vi "PAQ_FileRef_read_all_samples.vi"(8 "error in (no error)":errorcluster, 11 "refnum in":refnum<file>) -> (0 "error out":errorcluster, 1 "data":T1, 2 "Fetched samples":i32, 3 "refnum out":refnum<file>)   [LabVIEW 2020, in "Sgraph_lib_V1.lvlib" / "DBAL-BIN.lvclass"]
doc: "Read all samples from one PAQ file based on a file reference.\nThis VI will leave the file open, with the pointer right where the first data should be saved.\nPurpose is to replace the whole file content with a new data portion added.\nIn this way a file concatenate action without segmentation is performed."
uses:
  DBAL-BIN.lvclass
  controls/BIN/BINdata.ctl
panel:
  out "TAGs":string[](array[string])
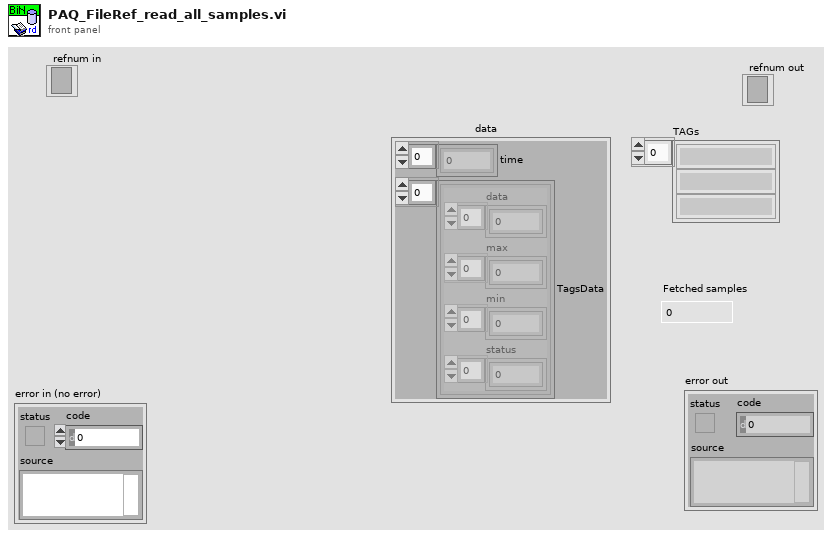
[diagram p1: front panel]
types:
  T1 = typedef "Sgraph_lib_V1.lvlib/DBAL-BIN.lvclass/BINdata.ctl" = cluster{"time":dbl[], "TagsData":cluster{"data":dbl[], "max":dbl[], "min":dbl[], "status":u32[]}[]}
  T2 = cluster{"data":dbl[], "max":dbl[], "min":dbl[], "status":u32[]}[]
  T3 = cluster{"data":dbl[], "max":dbl[], "min":dbl[], "status":u32[]}
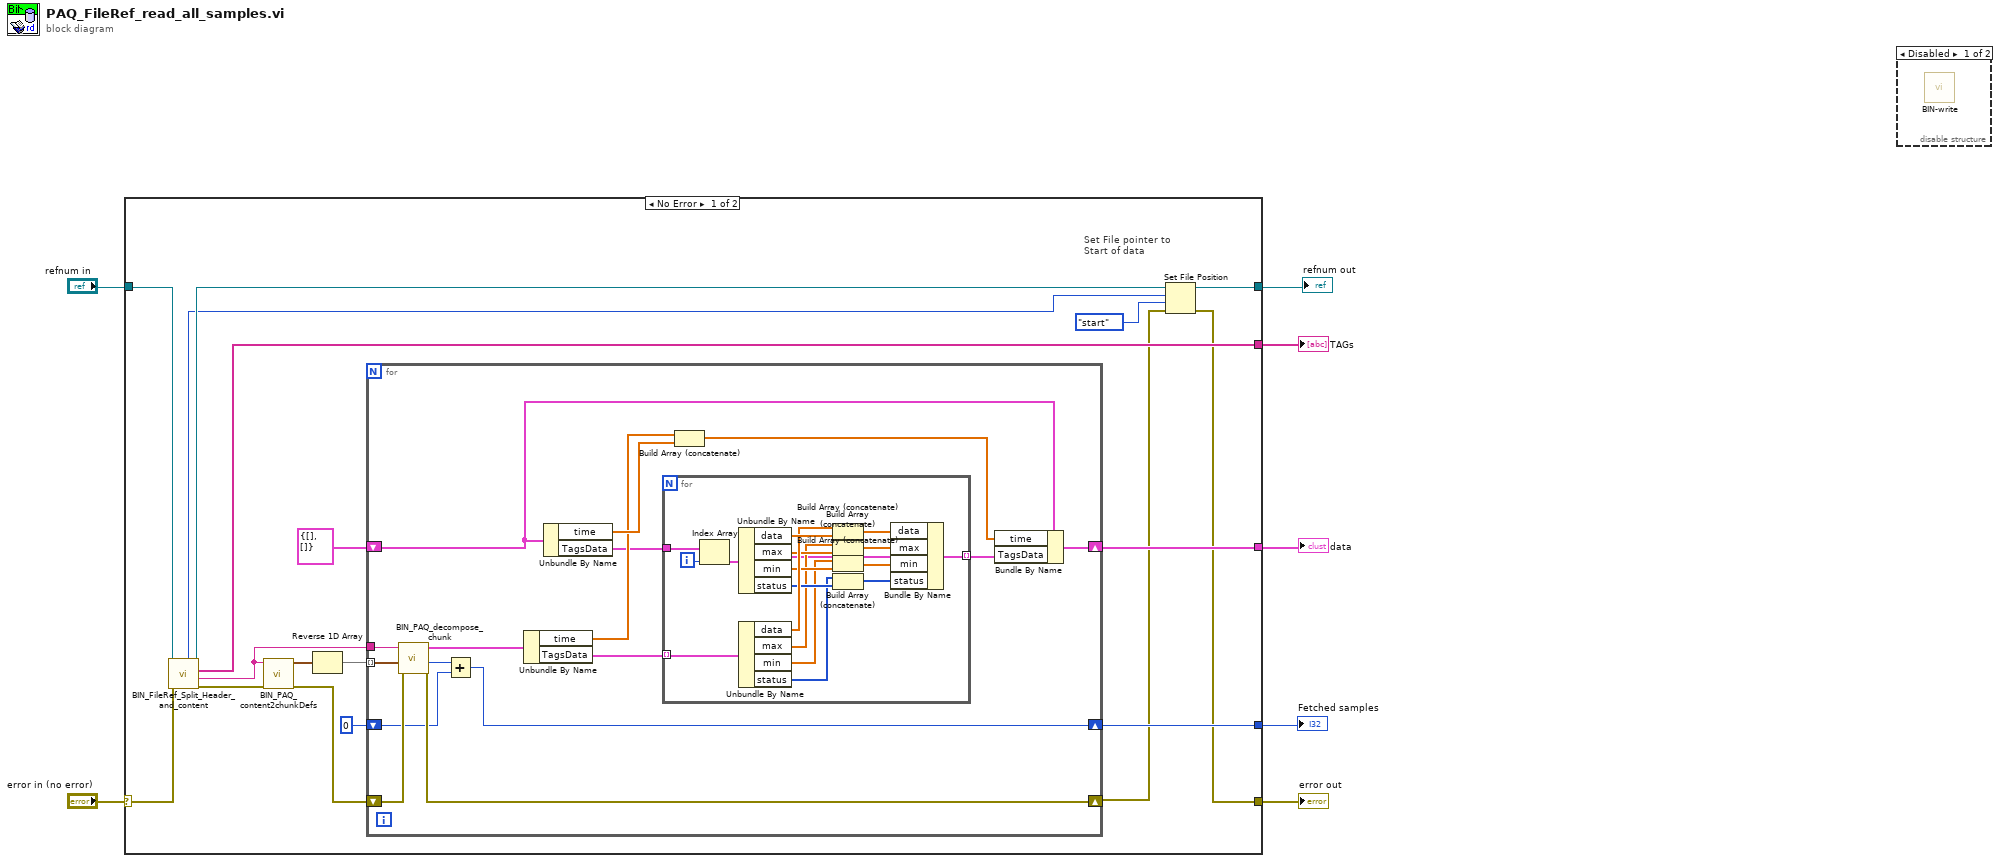
[diagram p0: block diagram]
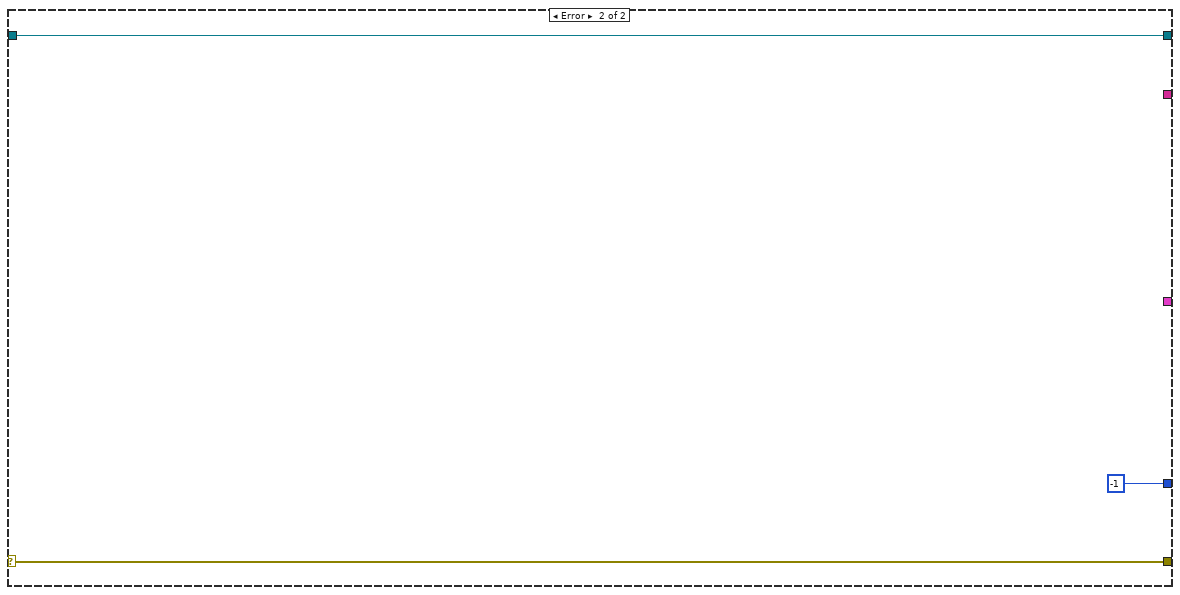
[diagram p3: hidden frame]
diagram:
  n1 = case shown="No Error" "error in (no error)" {
    selector: "error in (no error)" -> [w18 w61]
    tunnel: [w9 w61] -> w6
    tunnel: [w20 -1 ("Samples size")] -> w3
    tunnel: [w19 _] -> w5
    tunnel: [w15 _] -> w4
    tunnel: "refnum in" -> [w14 w59]
    tunnel: [w11 w59] -> w1
    frame No Error {
      # "Set File pointer to\nStart of data"
      n2 = call "BIN_FileRef_Split_Header_and_content.vi"("error in"=w18, "refnum in"=w14) -> ("error out"=w17:errorcluster, "Content"=w16:string, "TAGs"=w15:string[], "refnum out"=w12:refnum<file>, "start of data"=w8:i64)  [unwired: 5 in]
      n3 = call "BIN_PAQ_content2chunkDefs.vi"("error in (no error)"=w17, "Content"=w16) -> ("error out"=w25:errorcluster, "Data segments"=w24:cluster{"Offset":u32, "Size":u32}[])  [unwired: 8 in]
      n4 = Reverse 1D Array(array=w24) -> (reversed array=w23:cluster{"Offset":u32, "Size":u32}[])
      n5 = for {
        tunnel: w23 -> [w41] mode=indexing
        tunnel: w16 -> [w40]
        shift-right: [w38] -> w10
        shift-left: w25 -> [w39]
        shift-right: [w26] -> w20
        shift-left: 0 ("Samples size") -> [w28]
        shift-right: [w35] -> w19
        shift-left: T1 {"time"=[], "TagsData"=[]} ("PAQ_data") -> [w37]
        n6 = call "BIN_PAQ_decompose_chunk.vi"("error in (no error)"=w39, "Offset"=w41, "Content"=w40) -> ("error out"=w38:errorcluster, "Samples size"=w29:i32, "PAQ_data"=w36:T1)  [unwired: 6 in]
        n7 = Add(x=w29, y=w28) -> (x+y=w26:i32)
        n8 = Unbundle By Name(w36) -> ("time"=w33:dbl[], "TagsData"=w32:T2)
        n9 = Unbundle By Name(w37) -> ("time"=w34:dbl[], "TagsData"=w31:T2)
        n10 = for {
          tunnel: w32 -> [w56] mode=indexing
          tunnel: w31 -> [w58]
          tunnel: [w46] -> w30 mode=indexing
          i -> [w57]
          n11 = Index Array(array=w58, index=w57) -> (element=w47:T3)
          n12 = Unbundle By Name(w47) -> ("data"=w55:dbl[], "max"=w53:dbl[], "min"=w52:dbl[], "status"=w51:u32[])
          n13 = Unbundle By Name(w56) -> ("data"=w54:dbl[], "max"=w48:dbl[], "min"=w49:dbl[], "status"=w50:u32[])
          n14 = Build Array (concatenate)(w54, w55) -> (w43:dbl[])
          n15 = Build Array (concatenate)(w48, w53) -> (w44:dbl[])
          n16 = Build Array (concatenate)(w49, w52) -> (w45:dbl[])
          n17 = Build Array (concatenate)(w50, w51) -> (w42:u32[])
          n18 = Bundle By Name(cluster=w47, "data"=w43, "max"=w44, "min"=w45, "status"=w42) -> (w46:T3)
        }
        n19 = Build Array (concatenate)(w33, w34) -> (w27:dbl[])
        n20 = Bundle By Name(cluster=w37, "time"=w27, "TagsData"=w30) -> (w35:T1)
      }
      n21 = Set File Position(offset (in bytes) (0)=w8, refnum=w12, from (0:start)=enum16{"start", "end", "current"}."start", error in=w10) -> (refnum out=w11:refnum<file>, error out=w9:errorcluster)
    }
    frame Error {
    }
  }
  "error out" <- w6
  "Fetched samples" <- w3
  "TAGs" <- w4
  "data" <- w5
  "refnum out" <- w1
  n22 = disable-structure shown="Disabled" {
    frame Disabled {
      n23 = call "BIN-write.vi"() -> ()  [unwired: 9 in, 3 out]
    }
    frame Enabled {
    }
  }
